vi "Swerve Math.vi"(9 "Yaw":dbl=-5.71, 10 "Rot. Point Y":dbl, 11 "Rot. Point X":dbl) -> (3 "Swerve Math Ouput":dbl[](array[numeric])=[0.0, 0.0, 0.0, 0.0, 0.0, 10.75, 16.677080080157918, 12.75])   [LabVIEW 2018]
uses:
  Drive Train Global.vi
  Robot Information/Robot Information Global.vi
  <vilib>/addons/control/pid/pid.llb/PID (DBL).vi
  <vilib>/addons/control/pid/NI_PID_pid.lvlib
panel:
  in  "PID gains":T1={"proportional gain (Kc)"=0.03, "integral time (Ti, min)"=0.0, "derivative time (Td, min)"=0.0} {"derivative time (Td, min)" format="%.3f"; "integral time (Ti, min)" format="%.3f"; "proportional gain (Kc)" format="%.3f"}
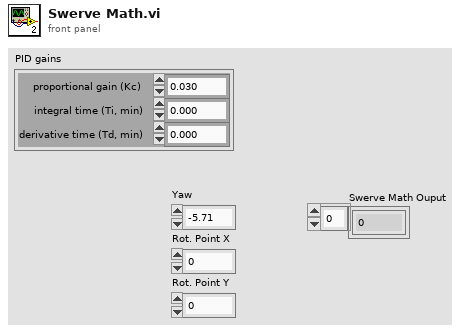
[diagram p1: front panel]
types:
  T1 = cluster{"proportional gain (Kc)":dbl, "integral time (Ti, min)":dbl, "derivative time (Td, min)":dbl}
  T2 = cluster{"Rollover":dbl, "Yaw":dbl, "Cont Yaw":dbl}
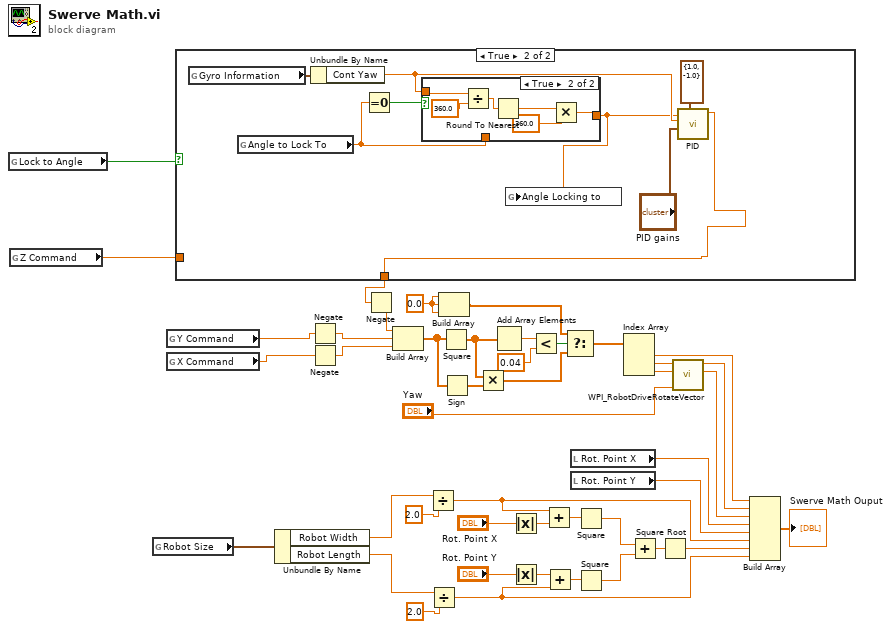
[diagram p0: block diagram]
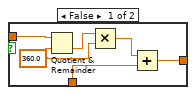
[diagram p3: hidden frame]
diagram:
  w15 = 0.0 ("element")
  n1 = global read "Drive Train Global.vi" "Lock to Angle"() -> (w7:bool)
  n2 = global read "Drive Train Global.vi" "Z Command"() -> (w8:dbl)
  n3 = global read "Robot Information Global.vi" "Robot Size"() -> (w22:cluster{"Robot Width":dbl, "Robot Length":dbl})
  n4 = global read "Drive Train Global.vi" "Y Command"() -> (w5:dbl)
  n5 = global read "Drive Train Global.vi" "X Command"() -> (w3:dbl)
  n6 = case shown="True" w7 {
    tunnel: [w45 w46] -> w1
    tunnel: w8 -> [w45 _]
    frame False {
    }
    frame True {
      n7 = global read "Drive Train Global.vi" "Gyro Information"() -> (w53:T2)
      n8 = global read "Drive Train Global.vi" "Angle to Lock To"() -> (w48:dbl)
      n9 = Unbundle By Name(w53) -> ("Cont Yaw"=w50:dbl)
      n10 = Equal To 0?(x=w48) -> (x = 0?=w47:bool)
      n11 = case shown="True" w47 {
        tunnel: w50 -> [w59 w65]
        tunnel: w48 -> [w58 _]
        tunnel: [w57 w60] -> w49
        frame False {
          w55 = 360.0 ("y")
          n12 = Quotient & Remainder(x=w59, y=w55) -> (floor(x/y)=w56:dbl)  [unwired: 1 out]
          n13 = Multiply(x=w56, y=w55) -> (x*y=w54:dbl)
          n14 = Add(x=w54, y=w58) -> (x+y=w57:dbl)
        }
        frame True {
          n15 = Divide(x=w65, y=360.0) -> (x/y=w63:dbl)
          n16 = Round To Nearest(number=w63) -> (nearest integer value=w62:dbl)
          n17 = Multiply(x=w62, y=360.0) -> (x*y=w60:dbl)
        }
      }
      n18 = global write "Drive Train Global.vi" "Angle Locking to"(w49) -> ()
      n19 = call-poly <vilib>:"PID.vi"("output range"=cluster{"output high":dbl, "output low":dbl} {"output high"=1.0, "output low"=-1.0}, "PID gains"="PID gains", "process variable"=w50, "setpoint"=w49) -> ("output"=w46:dbl)  [unwired: 6 in, 1 out]
    }
  }
  n20 = Unbundle By Name(w22) -> ("Robot Width"=w20:dbl, "Robot Length"=w21:dbl)
  n21 = Negate(x=w5) -> (-x=w6:dbl)
  n22 = Negate(x=w3) -> (-x=w4:dbl)
  n23 = Negate(x=w1) -> (-x=w2:dbl)
  n24 = Build Array(w2, w6, w4) -> (w11:dbl[])
  n25 = Divide(x=w20, y=2.0) -> (x/y=w30:dbl)
  n26 = Divide(x=w21, y=2.0) -> (x/y=w28:dbl)
  n27 = Build Array(w15, w15, w15) -> (w16:dbl[])
  n28 = Square(x=w11) -> (x^2=w13:dbl[])
  n29 = Sign(1:w11) -> (0:w14:dbl[])
  n30 = Multiply(x=w13, y=w14) -> (x*y=w12:dbl[])
  n31 = Add Array Elements(numeric array=w13) -> (sum=w19:dbl)
  n32 = Absolute Value(x="Rot. Point X") -> (abs(x)=w44:dbl)
  n33 = Absolute Value(x="Rot. Point Y") -> (abs(x)=w42:dbl)
  n34 = Less?(x=w19, y=0.04 ("x")) -> (x < y?=w17:bool)
  n35 = Add(x=w30, y=w44) -> (x+y=w43:dbl)
  n36 = Add(x=w42, y=w28) -> (x+y=w41:dbl)
  n37 = Select(t=w16, s=w17, f=w12) -> (s? t:f=w26:dbl[])
  n38 = local read "Rot. Point X"() -> (w32:dbl)
  n39 = local read "Rot. Point Y"() -> (w31:dbl)
  n40 = Square(x=w43) -> (x^2=w39:dbl)
  n41 = Square(x=w41) -> (x^2=w40:dbl)
  n42 = Index Array(array=w26) -> (element #1=w24:dbl, element #2=w27:dbl, element #3=w33:dbl)  [unwired: 3 in]
  n43 = Add(x=w39, y=w40) -> (x+y=w38:dbl)
  n44 = Square Root(x=w38) -> (sqrt(x)=w29:dbl)
  n45 = call <vilib>:"WPI_RobotDriveRotateVector.vi"("Angle"="Yaw", "X"=w33, "Y"=w27) -> ("X'"=w25:dbl, "Y'"=w23:dbl)  [unwired: 7 out]
  n46 = Build Array(w24, w23, w25, w32, w31, w30, w29, w28) -> (→"Swerve Math Ouput":dbl[])
